vi "Sum_Spectrum_XY.vi"(1 "array":T1) -> (0 "Array":dbl[][](array[numeric]))   [LabVIEW 2020]
uses:
  Control.ctl
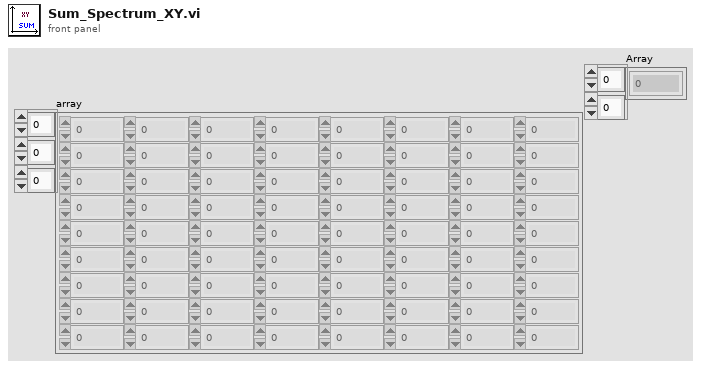
[diagram p1: front panel]
types:
  T1 = typedef "Control.ctl" = dbl[][][]
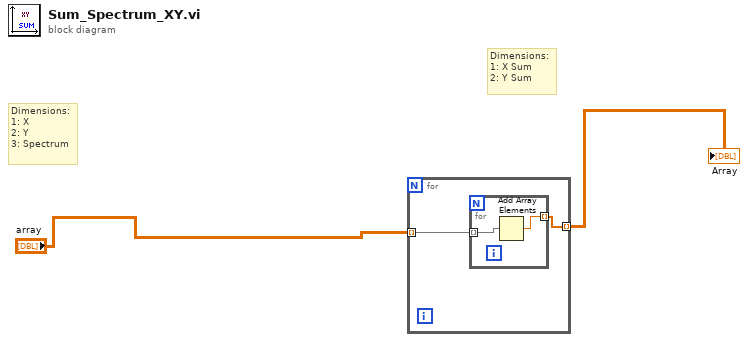
[diagram p0: block diagram]
diagram:
  # "Dimensions:\n1: X Sum\n2: Y Sum"
  # "Dimensions:\n1: X\n2: Y\n3: Spectrum"
  n1 = for {
    tunnel: "array" -> [w4] mode=indexing
    tunnel: [w3] -> w2 mode=indexing
    n2 = for {
      tunnel: [w6] -> w3 mode=indexing
      tunnel: w4 -> [w5] mode=indexing
      n3 = Add Array Elements(numeric array=w5) -> (sum=w6:dbl)
    }
  }
  "Array" <- w2
